vi "ConnectR.vi"(0 "VISA resource name":refnum<visa-resource-name>, 5 "error in":errorcluster) -> (14 "RBD9103":T1, 19 "error out":errorcluster)   [LabVIEW 2018]
uses:
  RBD9103.ctl
  GenericDataEvent/GenericEvent.ctl
  <vilib>/Instr/_visa.llb/VISA Configure Serial Port (Instr).vi
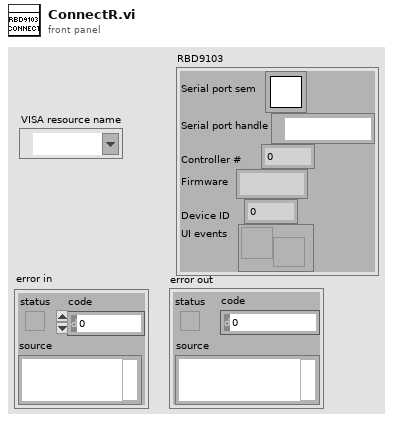
[diagram p1: front panel]
types:
  T1 = typedef "RBD9103.ctl" = cluster{"Serial port sem":T2, "Serial port handle":refnum<visa-resource-name>, "Controller #":u8, "Firmware":string, "Device ID":i32, "UI events":T3}
  T2 = typedef "Semaphore RefNum" = refnum<k1>
  T3 = typedef "GenericEvent.ctl" = refnum<user-event>
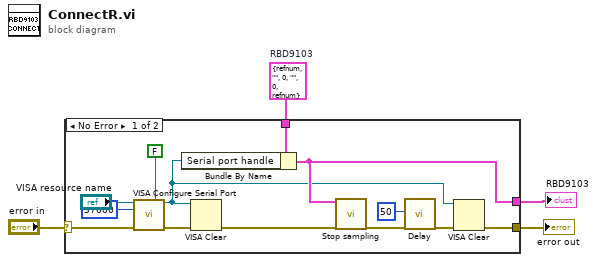
[diagram p0: block diagram]
diagram:
  w2 = T1 {"Serial port sem"=refnum, "Serial port handle"="", "Controller #"=0, "Firmware"="", "Device ID"=0, "UI events"=refnum}  # RBD9103
  n1 = case shown="No Error" "error in" {
    selector: "error in" -> [w10 w19]
    tunnel: [w6 w19] -> w3
    tunnel: [w13 w18] -> w1
    tunnel: w2 -> [w17 w18]
    frame No Error {
      n2 = call-poly "VISA Configure Serial Port"("VISA resource name"="VISA resource name", "Enable Termination\nChar (T)"=FALSE ("Enable Termination\nChar (T)"), "baud rate (9600)"=u32 57600, "error in (no error)"=w10) -> ("VISA resource name out"=w5:refnum<visa-resource-name>, "error out"=w9:errorcluster)  [unwired: 10 in]
      n3 = Bundle By Name(cluster=w17, "Serial port handle"=w5) -> (w13:T1)
      n4 = VISA Clear(VISA resource name=w5, error in (no error)=w9) -> (error out=w8:errorcluster)  [unwired: 1 out]
      n5 = call "Stop sampling.vi"("RBD9103"=w13, "error in"=w8) -> ("error out"=w12:errorcluster)  [unwired: 16 in, 1 out]
      n6 = call "Delay.vi"("Delay, ms"=u32 50, "error in"=w12) -> ("error out"=w7:errorcluster)  [unwired: 17 in]
      n7 = VISA Clear(VISA resource name=w5, error in (no error)=w7) -> (error out=w6:errorcluster)  [unwired: 1 out]
    }
    frame Error {
    }
  }
  "error out" <- w3
  "RBD9103" <- w1
